vi "Initialize.vi"(8 "error in (no error)":errorcluster, 9 "Npts":i32=-1, 10 "Owner":string, 11 "SigMan in":refnum<class "SignalManager.lvclass">) -> (0 "error out":errorcluster, 3 "SigMan out":refnum<class "SignalManager.lvclass">)   [LabVIEW 2015, in "SignalManager.lvclass"]
uses:
  SignalManager.lvclass
  SignalManager.lvclass/SignalManager.ctl
  Channel/Channel.lvclass/Channel.ctl
  Channel/Read Destination.vi
  Channel/Channel.lvclass
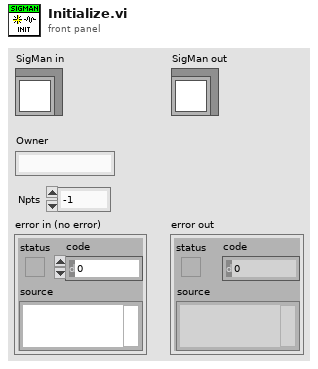
[diagram p1: front panel]
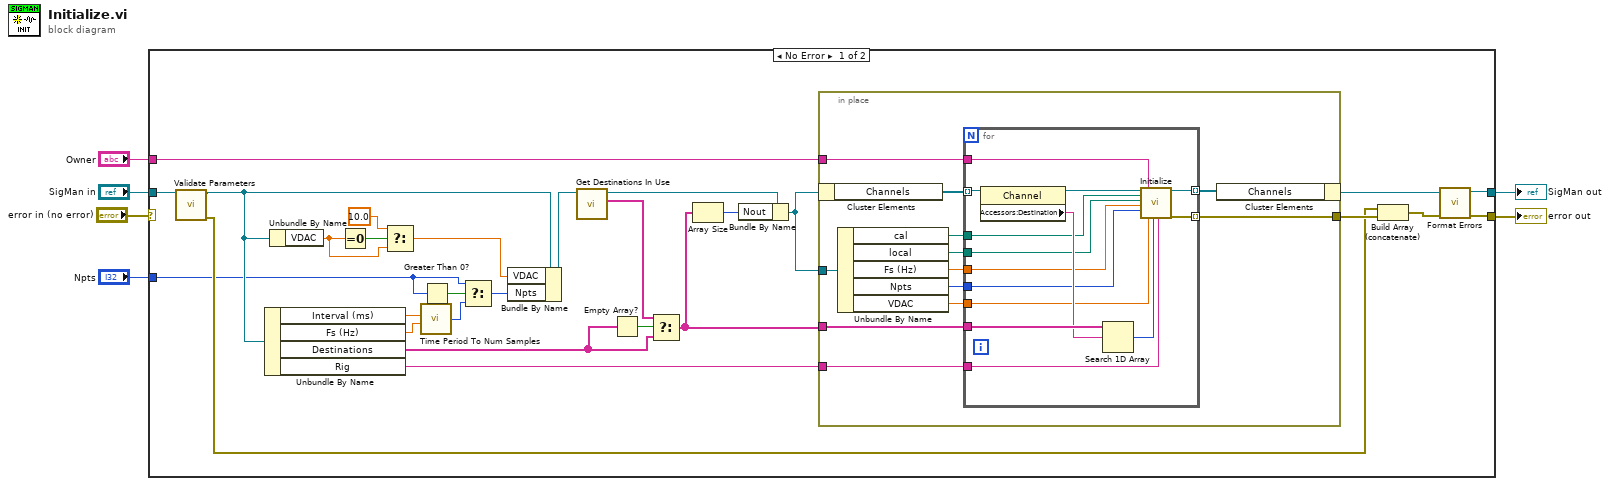
[diagram p0: block diagram]
diagram:
  n1 = case shown="No Error" "error in (no error)" {
    selector: "error in (no error)" -> [_ w62]
    tunnel: [w30 w62] -> w5
    tunnel: [w31 w61] -> w3
    tunnel: "SigMan in" -> [w34 w61]
    tunnel: "Owner" -> [w12 _]
    tunnel: "Npts" -> [w8 _]
    frame No Error {
      n2 = call "Validate Parameters.vi"("SigMan in"=w34) -> ("error out"=w14:errorcluster, "SigMan out"=w33:refnum<class "SignalManager.lvclass">)  [unwired: 9 in]
      n3 = Unbundle By Name(w33) -> ("Interval (ms)"=w27:dbl, "Fs (Hz)"=w26:dbl, "Destinations"=w21:string[], "Rig"=w7:string)
      n4 = Unbundle By Name(w33) -> ("VDAC"=w18:dbl)
      n5 = Equal To 0?(x=w18) -> (x = 0?=w20:bool)
      n6 = Select(t=10.0, s=w20, f=w18) -> (s? t:f=w16:dbl)
      n7 = call "Time Period To Num Samples.vi"("Duration (ms)"=w27, "Sampling rate (Hz)"=w26) -> ("Samples"=w10:i32)  [unwired: 5 in]
      n8 = Greater Than 0?(x=w8) -> (x > 0?=w11:bool)
      n9 = Select(t=w8, s=w11, f=w10) -> (s? t:f=w9:i32)
      n10 = Bundle By Name(cluster=w33, "VDAC"=w16, "Npts"=w9) -> (w28:refnum<class "SignalManager.lvclass">)
      n11 = call "Get Destinations In Use.vi"("SigMan in"=w28) -> ("Destinations in use"=w22:string[], "SigMan out"=w17:refnum<class "SignalManager.lvclass">)  [unwired: 8 in, 1 out]
      n12 = Empty Array?(array=w21) -> (empty?=w23:bool)
      n13 = Select(t=w22, s=w23, f=w21) -> (s? t:f=w13:string[])
      n14 = Array Size(array=w13) -> (size(s)=w25:i32)
      n15 = Bundle By Name(cluster=w17, "Nout"=w25) -> (w24:refnum<class "SignalManager.lvclass">)
      n16 = in-place {
        in-place-border: w13 -> [w44]
        in-place-border: w24 -> [w45]
        in-place-border: [w39] -> w29
        in-place-border: w12 -> [w36]
        in-place-border: w7 -> [w35]
        n17 = in-place-cluster #1(w24) -> ("Channels"=w46:refnum<class "Channel.lvclass">[])
        n18 = Unbundle By Name(w45) -> ("cal"=w38:path, "local"=w42:path, "Fs (Hz)"=w41:dbl, "Npts"=w40:i32, "VDAC"=w37:dbl)
        n19 = for {
          tunnel: w46 -> [w60] mode=indexing
          tunnel: w44 -> [w59]
          tunnel: [w56] -> w43 mode=indexing
          tunnel: w42 -> [w52]
          tunnel: w41 -> [w55]
          tunnel: w40 -> [w54]
          tunnel: [w53] -> w39 mode=indexing
          tunnel: w38 -> [w51]
          tunnel: w37 -> [w49]
          tunnel: w36 -> [w48]
          tunnel: w35 -> [w47]
          n20 = property class="Channel"(reference=w60) -> (reference out=w57:refnum<class "Channel.lvclass">, "Accessors:Destination"=w58:string)  [unwired: 1 in, 1 out]
          n21 = Search 1D Array(1D array=w59, element=w58) -> (index of element=w50:i32)  [unwired: 1 in]
          n22 = call "Initialize.vi"("Channel in"=w57, "Calibration folder"=w51, "Local folder"=w52, "Fs (Hz)"=w55, "Npts"=w54, "SigMan Name"=w48, "Vmax"=w49, "Number"=w50, "Rig"=w47) -> ("Channel out"=w56:refnum<class "Channel.lvclass">, "error out"=w53:errorcluster)  [unwired: 9 in]
        }
        n23 = in-place-cluster #1("Channels"=w43) -> (w32:refnum<class "SignalManager.lvclass">)
      }
      n24 = Build Array (concatenate)(w14, w29) -> (w15:errorcluster[])
      n25 = call "Format Errors.vi"("error in (no error)"=w15, "SigMan in"=w32) -> ("error out"=w30:errorcluster, "SigMan out"=w31:refnum<class "SignalManager.lvclass">)  [unwired: 8 in]
    }
    frame Error {
    }
  }
  "error out" <- w5
  "SigMan out" <- w3
